vi "sortDependencies.vi"(8 "error in (no error)":errorcluster, 10 "Dependency Paths":path[](array[path]), 11 "Dependency in":refnum<class "Dependency.lvclass">) -> (0 "error out":errorcluster, 1 "ControlDependencyPaths":path[](array[path]), 2 "VIDependencyPaths":path[](array[path]), 3 "Dependency out":refnum<class "Dependency.lvclass">)   [LabVIEW 2016, in "Dependency.lvclass"]
uses:
  Dependency.lvclass
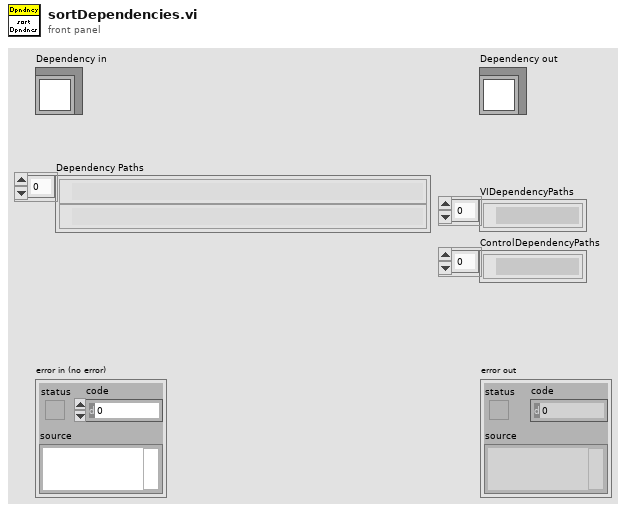
[diagram p1: front panel]
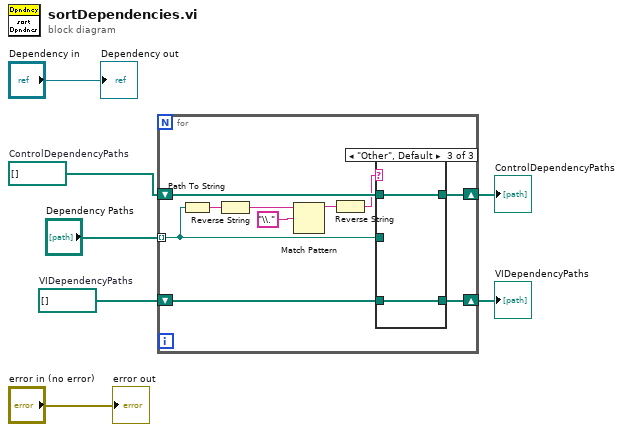
[diagram p0: block diagram]
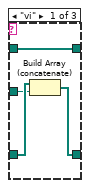
[diagram p2: hidden frame]
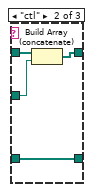
[diagram p3: hidden frame]
diagram:
  w3 = path[] []  # ControlDependencyPaths
  w4 = path[] []  # VIDependencyPaths
  n1 = for {
    tunnel: "Dependency Paths" -> [w15] mode=indexing
    shift-right: [w14] -> w1
    shift-left: w4 -> [w16]
    shift-right: [w12] -> w2
    shift-left: w3 -> [w13]
    n2 = Path To String(path=w15) -> (string=w11:string)
    n3 = Reverse String(1:w11) -> (0:w10:string)
    n4 = Match Pattern(string=w10, regular expression="\\.") -> (before substring=w9:string)  [unwired: 1 in, 3 out]
    n5 = Reverse String(1:w9) -> (0:w8:string)
    n6 = case shown="\"Other\", Default" w8 {
      tunnel: w16 -> [w21 w22 w26]
      tunnel: w15 -> [w20 w23 _]
      tunnel: [w19 w22 w26] -> w14
      tunnel: w13 -> [w18 w25 w27]
      tunnel: [w18 w24 w27] -> w12
      frame "vi" {
        n7 = Build Array (concatenate)(w21, w20) -> (w19:path[])
      }
      frame "ctl" {
        n8 = Build Array (concatenate)(w25, w23) -> (w24:path[])
      }
      frame "Other", Default {
      }
    }
  }
  "VIDependencyPaths" <- w1
  "ControlDependencyPaths" <- w2
  "error out" <- "error in (no error)"
  "Dependency out" <- "Dependency in"
